vi "Register for Events.vi"(8 "Error In":errorcluster, 11 "Panel Actor in":refnum<class "Panel Actor.lvclass">) -> (0 "Error Out":errorcluster, 2 "Panel Helper":refnum<class "Panel Helper.lvclass">, 3 "Panel Actor out":refnum<class "Panel Actor.lvclass">, 5 "Pnl Actor":refnum<event-registration> caption="Panel Actor Events", 7 "Self Enqueuer":refnum<class "Message Enqueuer.lvclass">)   [LabVIEW 2017, in "MGI-Panel Actor.lvlib" / "Panel Actor.lvclass"]
doc: "Registers for the Actor Events. The self Enqueuer is returned for convenience.\n\nNote: This VI will register for events even on error in. This is to ensure your Event Handler loop will get the stop even event if an error has been generated.\n\n<B>Panel Actor In:</B> Panel Actor object\n<B>Offset:</B> Input Offset object.\n<B>Self Enqueuer:</B> Self Enqueuer object.\n<B>Panel Actor Events:</B> Event Registration refnum for panel-defined user events.\n<B>Error In:</B> Describes error conditions that occur before this node runs.\n\n<B>Panel Actor Out:</B> Panel Actor object.\n<B>Error Out:</B> Contains error information.\n----\nCopyright: MGI 2018\nAuthor: Derek Trepanier"
uses:
  Panel Actor.lvclass
  C:/Program Files (x86)/National Instruments/LabVIEW 2017/vi.lib/ActorFramework/Actor/Actor.lvclass
  <vilib>/ActorFramework/Message Enqueuer/Message Enqueuer.lvclass
  panel-manager/Source/Panel Helper/Panel Events.ctl
  panel-manager/Source/Panel Helper/Events.ctl
  panel-manager/Source/Panel Helper/Panel Helper.lvclass
  Panel Actor.lvclass/Panel Actor.ctl
  <vilib>/ActorFramework/Actor/Actor.lvclass/Actor.ctl
  <vilib>/ActorFramework/Message Enqueuer/Message Enqueuer.lvclass/Message Enqueuer.ctl
  <vilib>/ActorFramework/Message Enqueuer/Init from Existing Queue.vi
  <vilib>/ActorFramework/Actor/Actor.lvclass
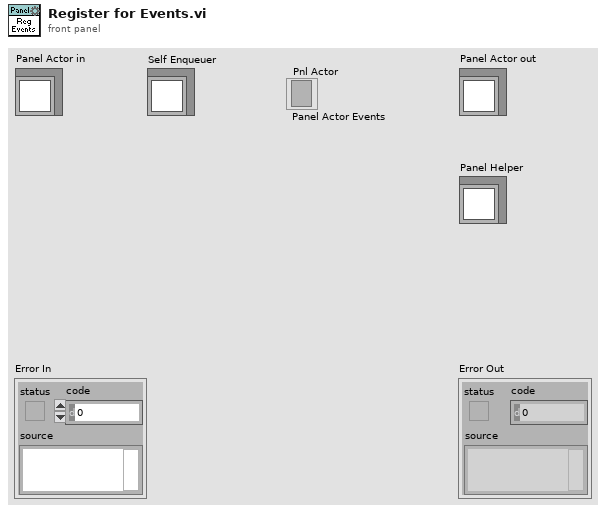
[diagram p1: front panel]
types:
  T1 = cluster{"Initialized":refnum<user-event>, "Stopped":refnum<user-event>}
  T2 = typedef "MGI-Panel Manager.lvlib/Panel Helper.lvclass/Panel Events.ctl" = cluster{"My Panel":refnum<user-event>, "Top Level Initialized":refnum<user-event>}
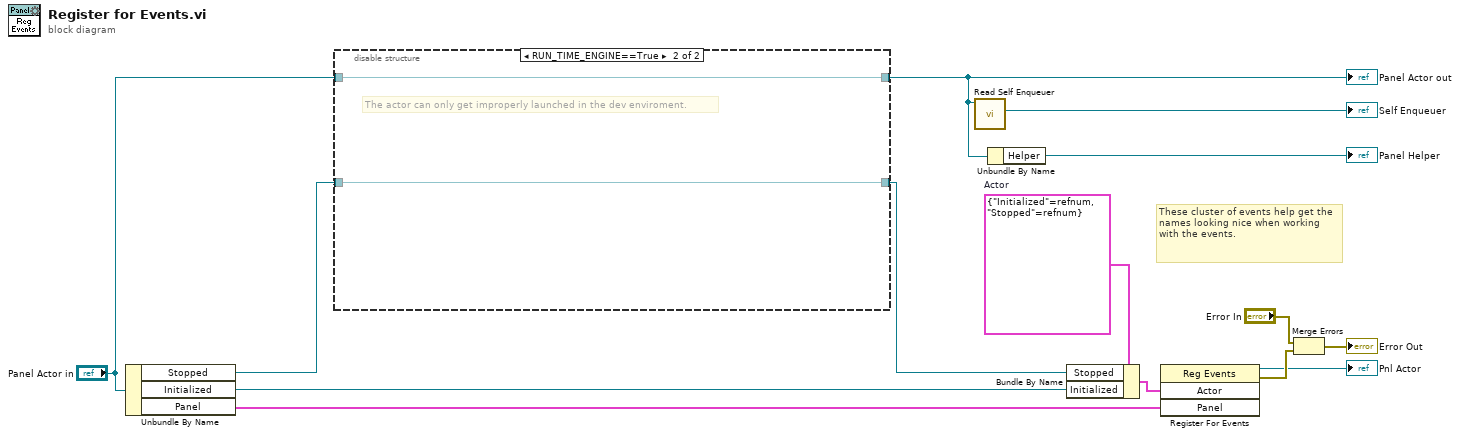
[diagram p0: block diagram]
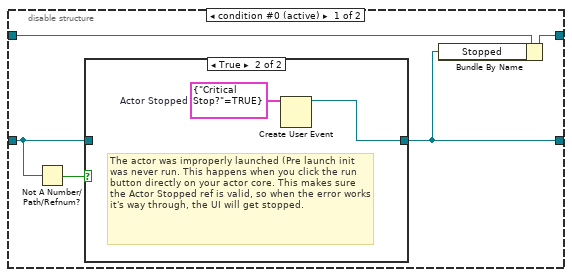
[diagram p2: hidden frame]
diagram:
  w8 = T1 {"Initialized"=refnum, "Stopped"=refnum}  # Actor
  # "These cluster of events help get the names looking nice when working with the events."
  n1 = Unbundle By Name("Panel Actor in") -> ("Stopped"=w10:refnum<user-event>, "Initialized"=w5:refnum<user-event>, "Panel"=w4:T2)
  n2 = disable-structure shown="RUN_TIME_ENGINE==True" {
    disable-tunnel: w10 -> [w18 w24]
    disable-tunnel: [w15 w24] -> w6
    disable-tunnel: [w16 w23] -> w2
    disable-tunnel: "Panel Actor in" -> [w17 w23]
    frame condition #0 (active) {
      n3 = Not A Number/Path/Refnum?(number/path/refnum=w18) -> (NaN/Path/Refnum?=w19:bool)
      n4 = case shown="True" w19 {
        tunnel: w18 -> [w20 _]
        tunnel: [w20 w21] -> w15
        frame False {
        }
        frame True {
          w22 = cluster{"Critical Stop?":bool} {"Critical Stop?"=TRUE}  # Actor Stopped
          # "The actor was improperly launched (Pre launch init was never run. This happens when you click the run button directly on your actor core. This makes sure the Actor Stopped ref is valid, so when the error works it's way through, the UI will get stopped."
          n5 = Create User Event(user event datatype=w22) -> (user event=w21:refnum<user-event>)  [unwired: 1 in, 1 out]
        }
      }
      n6 = Bundle By Name(cluster=w17, "Stopped"=w15) -> (w16:refnum<class "Panel Actor.lvclass">)
    }
    frame condition #1 {
      # "The actor can only get improperly launched in the dev enviroment."
    }
  }
  "Panel Actor out" <- w2
  n7 = call <vilib>:"Read Self Enqueuer.vi"("Actor"=w2) -> ("Self Enqueuer"=→"Self Enqueuer":refnum<class "Message Enqueuer.lvclass">)  [unwired: 10 in]
  n8 = Unbundle By Name(w2) -> ("Helper"=→"Panel Helper":refnum<class "Panel Helper.lvclass">)
  n9 = Bundle By Name(cluster=w8, "Stopped"=w6, "Initialized"=w5) -> (w7:T1)
  n10 = register-events(w7, w4) -> (reference out=→"Pnl Actor":refnum<event-registration>, error out=w11:errorcluster)  [unwired: 2 in]
  n11 = Merge Errors("Error In", w11) -> (→"Error Out":errorcluster)
